vi "QTrkReadTimestamp.vi"(10 "Use QTrk code?":bool, 11 "Image":T1) -> (3 "timestamp":u32)   [LabVIEW 2011]
uses:
  <vilib>/vision/Image Controls.llb/IMAQ Image.ctl
  QTrkDLL.vi
  <vilib>/vision/NI_Vision_Development_Module.lvlib
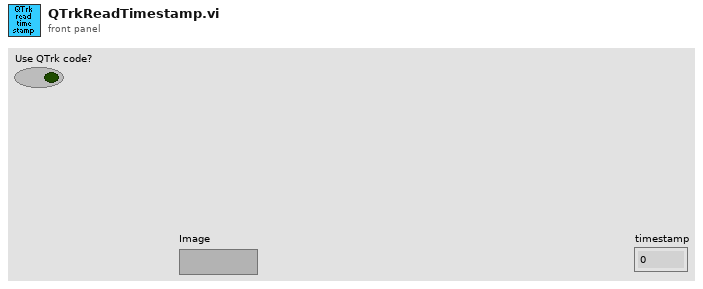
[diagram p1: front panel]
types:
  T1 = typedef "IMAQ Image.ctl" = refnum<image>
  T2 = enum32{"Map Pixel Pointer", "Unmap Pixel Pointer", "Get Pixels Infos"}
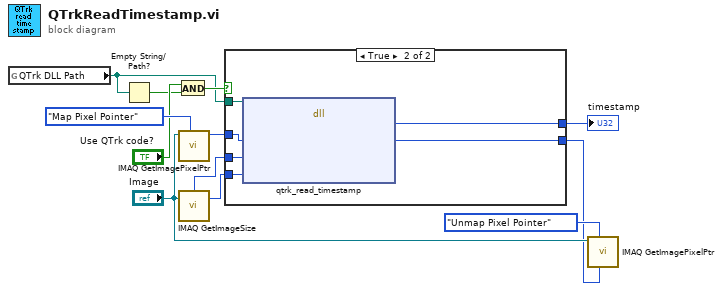
[diagram p0: block diagram]
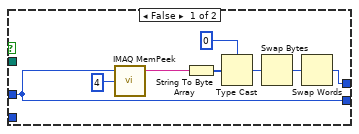
[diagram p2: hidden frame]
diagram:
  n1 = global read "QTrkDLL.vi" "QTrk DLL Path"() -> (w1:path)
  n2 = Empty String/Path?(string/path=w1) -> (empty?=w3:bool)
  n3 = And(x="Use QTrk code?", y=w3) -> (x .and. y?=w2:bool)
  n4 = call "IMAQ GetImagePixelPtr"("Function"=T2."Map Pixel Pointer", "Image"="Image") -> ("Pixel Pointer out"=w5:u64)  [unwired: 4 in, 5 out]
  n5 = call "IMAQ GetImageSize"("Image"="Image") -> ("Y Resolution"=w10:i32, "X Resolution"=w11:i32)  [unwired: 3 in, 1 out]
  n6 = case shown="True" w2 {
    tunnel: w11 -> [_ w26]
    tunnel: w10 -> [_ w25]
    tunnel: [w13 w24] -> w9
    tunnel: [w16 w23] -> w6
    tunnel: w5 -> [w16 w22]
    tunnel: w1 -> [_ w21]
    frame False {
      n7 = call "IMAQ MemPeek"("Bytes count"=4, "void*"=w16) -> ("Data string"=w18:string)  [unwired: 2 in, 1 out]
      n8 = String To Byte Array(string=w18) -> (unsigned byte array=w19:u8[])
      n9 = Type Cast(type=u32 0 ("unsigned 32bit integer"), x=w19) -> (*(type *) &x=w15:u32)
      n10 = Swap Bytes(anything=w15) -> (byte swapped=w14:u32)
      n11 = Swap Words(1:w14) -> (0:w13:u32)
    }
    frame True {
      n12 = dll-call lib="D:/jcnossen1/cudaqi-tracker/bin/jtrkcuda-labview.dll" fn="qtrk_read_timestamp"(path in=w21, "imageptr"=w22, "width"=w26, "height"=w25) -> ("timestamp"=w24:u32, "imageptr"=w23:u64)  [unwired: 4 in, 2 out]
    }
  }
  "timestamp" <- w9
  n13 = call "IMAQ GetImagePixelPtr"("Pixel Pointer in"=w6, "Function"=T2."Unmap Pixel Pointer", "Image"="Image") -> ()  [unwired: 3 in, 6 out]
